vi "Test_issueCommand_start.vi"(8 "error in (no error)":errorcluster, 11 "command_start_Ctl":T1={"private_rcvStamp"=0.0, "settingsToApply"="                                                                                                                                                                                                                                                                "}) -> (0 "error out":errorcluster, 2 "function return":i32, 3 "command_start_Ctl out":T1={"private_rcvStamp"=0.0, "settingsToApply"="                                                                                                                                                                                                                                                                "})   [LabVIEW 2018, in "SALLV_Test.lvlib"]
doc: "int Test_shm_issueCommand_startLV(Test_command_startLV *command_start_Ctl );"
uses:
  DataTypes/command_start.ctl
  SALLV_Test.lvlib
  SALLV_Test.so
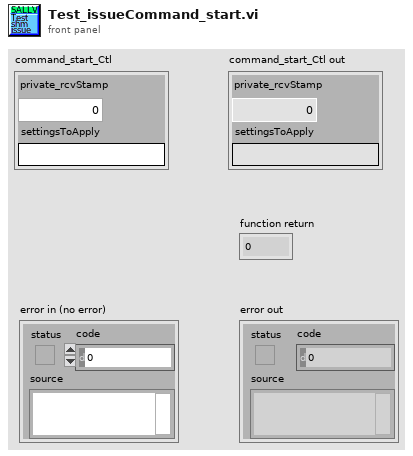
[diagram p1: front panel]
types:
  T1 = typedef "SALLV_Test.lvlib/command_start.ctl" = cluster{"private_rcvStamp":dbl, "settingsToApply":string}
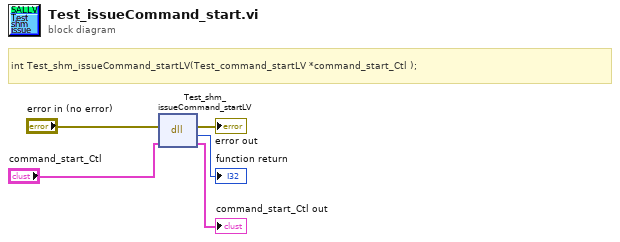
[diagram p0: block diagram]
diagram:
  # "int Test_shm_issueCommand_startLV(Test_command_startLV *command_start_Ctl );"
  n1 = dll-call lib="home/ttsai/Documents/salTestLabViewApi/SALLV_Test/SALLV_Test.*" fn="Test_shm_issueCommand_startLV"(error in="error in (no error)", "command_start_Ctl"="command_start_Ctl") -> (error out=→"error out":errorcluster, →"function return":i32, "command_start_Ctl"=→"command_start_Ctl out":T1)  [unwired: 2 in, 1 out]
